vi "YKMW100 Read Com Register.vi"(0 "VISA session":refnum<visa-resource-name>="MW100", 7 "Com Channel (C001)":string="C001", 9 "Timeout (25000)":u32=100, 11 "error in (no error)":errorcluster, 13 "Source (\"\")":string) -> (4 "dup VISA session":refnum<visa-resource-name>, 8 "Buffer Value":string, 15 "error out":errorcluster)   [LabVIEW 2009]
doc: "This VI sends the message. Then it returns the response."
panel:
  out "ENCRLF":string
  out "EACRLF":string
  out "Read Buffer":string
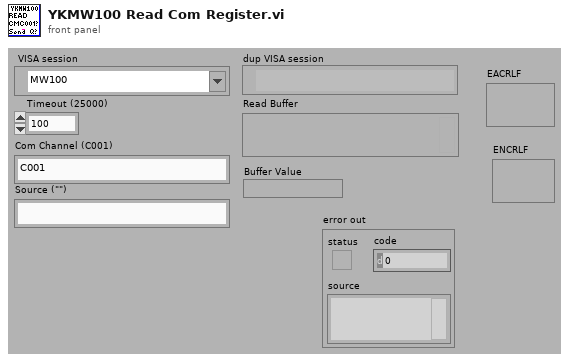
[diagram p1: front panel]
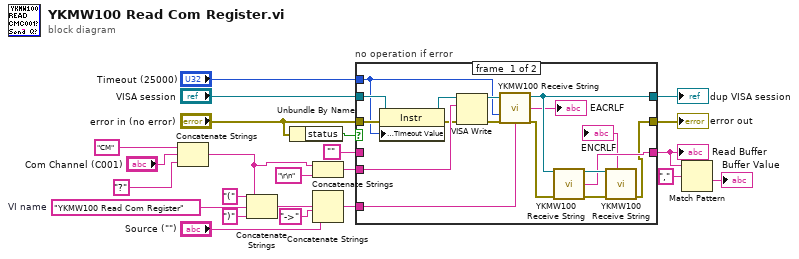
[diagram p0: block diagram]
diagram:
  w11 = "YKMW100 Read Com Register"  # VI name
  n1 = Concatenate Strings("CM" ("Send Message (\"\")"), "Com Channel (C001)", "?" ("Send Message (\"\")")) -> (w2:string)
  n2 = Concatenate Strings("(", w2, ")") -> (w12:string)
  n3 = Unbundle By Name("error in (no error)") -> ("status"=w18:bool)
  n4 = Concatenate Strings(w2, "\r\n") -> (w22:string)
  n5 = Concatenate Strings(w11, w12, "->", "Source (\"\")") -> (w17:string)
  n6 = case "no operation if error" shown="False" w18 {
    tunnel: "VISA session" -> [w37 w43]
    tunnel: w22 -> [w40 _]
    tunnel: [w29 w43] -> w10
    tunnel: [w26 w42] -> w23
    tunnel: "error in (no error)" -> [w39 w42]
    tunnel: w17 -> [w33 _]
    tunnel: "Timeout (25000)" -> [w32 _]
    tunnel: [w27 w41] -> w7
    tunnel: "" -> [_ w41]
    frame #0 {
      n7 = property class="Instr"(reference=w37, error in=w39, "General Settings:Timeout Value"=w32) -> (reference out=w36:refnum<visa-resource-name>, error out=w38:errorcluster)
      n8 = VISA Write(VISA resource name=w36, write buffer=w40, error in (no error)=w38) -> (VISA resource name out=w35:refnum<visa-resource-name>, error out=w34:errorcluster)  [unwired: 1 out]
      n9 = call "YKMW100 Receive String.vi"("VISA session"=w35, "Timeout (25000)"=w32, "error in (no error)"=w34, "Source (\"\")"=w33) -> ("dup VISA session"=w29:refnum<visa-resource-name>, "Read Buffer"=→"EACRLF":string, "error out"=w28:errorcluster)  [unwired: 9 in]
      n10 = call "YKMW100 Receive String.vi"("VISA session"=w29, "error in (no error)"=w28) -> ("dup VISA session"=w31:refnum<visa-resource-name>, "Read Buffer"=w27:string, "error out"=w30:errorcluster)  [unwired: 11 in]
      n11 = call "YKMW100 Receive String.vi"("VISA session"=w31, "error in (no error)"=w30) -> ("Read Buffer"=→"ENCRLF":string, "error out"=w26:errorcluster)  [unwired: 11 in, 1 out]
    }
    frame #1 {
    }
  }
  "error out" <- w23
  "dup VISA session" <- w10
  "Read Buffer" <- w7
  n12 = Match Pattern(string=w7, regular expression=",") -> (after substring=→"Buffer Value":string)  [unwired: 1 in, 3 out]
